vi "svx_Timebase Set Minimum Panel Size.vi"(7 "Facade VI":refnum<vi>, 9 "Graph Type":T1, 10 "Legend Width":i16, 11 "Legend Visible":bool=TRUE) -> ()   [LabVIEW 2017, in "SVX Timebase.xctl"]
uses:
  <vilib>/addons/_XControls/Timebase Plot/SVX Timebase.xctl
  <vilib>/addons/_XControls/Timebase Plot/subVIs/svx_Timebase Graph Types.ctl
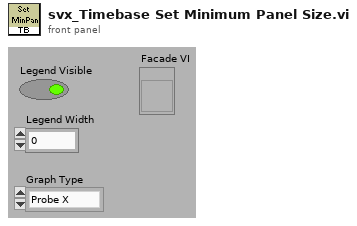
[diagram p1: front panel]
types:
  T1 = typedef "SVX Timebase.xctl/svx_Timebase Graph Types.ctl" = enum16{"Probe X", "Probe Y", "Probe X and Y"}
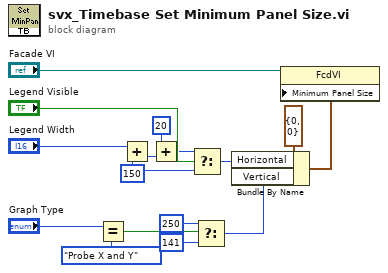
[diagram p0: block diagram]
diagram:
  w5 = i16 150 ("x")
  n1 = Equal?(x="Graph Type", y=svx_Timebase_Graph_Types."Probe X and Y" ("Graph Type")) -> (x = y?=w12:bool)
  n2 = Add(x="Legend Width", y=w5) -> (x+y=w2:i16)
  n3 = Add(x=i16 20, y=w2) -> (x+y=w3:i16)
  n4 = Select(t=w3, s="Legend Visible", f=w5) -> (s? t:f=w9:i16)
  n5 = Select(t=i16 250, s=w12, f=i16 141) -> (s? t:f=w8:i16)
  n6 = Bundle By Name(cluster=cluster{"Horizontal":i16, "Vertical":i16} {"Horizontal"=0, "Vertical"=0} ("Front Panel Window:Minimum Size"), "Horizontal"=w9, "Vertical"=w8) -> (w7:cluster{"Horizontal":i16, "Vertical":i16})
  n7 = property class="FcdVI"(reference="Facade VI", "Minimum Panel Size"=w7) -> ()  [unwired: 1 in, 2 out]
